vi "Z6_Beamline.Calc BL State.vi"(0 "i ref in":refnum<vi>, 5 "error in (nop error)":errorcluster) -> (14 "i ref out":refnum<vi>, 19 "error out":errorcluster)   [LabVIEW 2014, in "Z6_Beamline.lvlib"]
doc: "this VI calculates the global state of the beamline, writes the result to own attributes, and publishes it as service."
uses:
  Z6_Beamline.lvlib
  PH_BL-Master/PH_BL-Master.lvlib
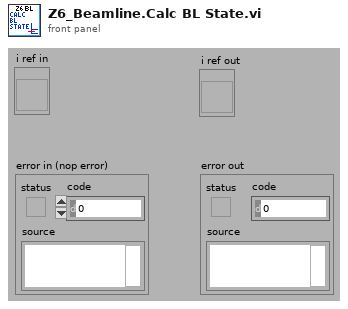
[diagram p1: front panel]
types:
  T1 = typedef "Z6_Beamline.lvlib/Z6_Beamline.i attribute.ctl" = cluster{"Subs ok GUI Refs":T2, "Refs BL Northtower":refnum<vi>[], "Refs BL Southtower":refnum<vi>[], "Refs BL 100TW COS":refnum<vi>[], "State Subsystems":cluster{"Northtower":bool, "Southtower":bool, "Frontends":bool, "100TW COS":bool}, "Z6 Beamline Status Subscriber Information":T3, "Color State PHELIX":i16}
  T2 = typedef "Z6_Beamline.lvlib/Z6_Beamline.Subsystem ok GUI Refs.ctl" = cluster{"Northtower ok":refnum<vi>, "Southtower ok":refnum<vi>, "Frontends ok":refnum<vi>, "100TW COS ok":refnum<vi>}
  T3 = typedef "Z6_Beamline.lvlib/Z6_Beamline.Status Subscriber Information.ctl" = cluster{"BL Z6 Shutter":T4, "CH 10":T4, "CH 11":T4, "ST Flip Cam":T4, "ST Flip DB":T4, "BL Z6 Dump":T4}
  T4 = typedef "PH_BL-Master.lvlib/PH_BL-Master.Status Subscriber Information.ctl" = cluster{"Index of element":i32, "Attributeset":T5}
  T5 = typedef "PH_BL-Master.lvlib/PH_BL-Master.Attribute Set.ctl" = enum16{"Boolean Status Service Subscriber", "Picture Status Service Subscriber"}
  T6 = cluster{"Northtower":bool, "Southtower":bool, "Frontends":bool, "100TW COS":bool}
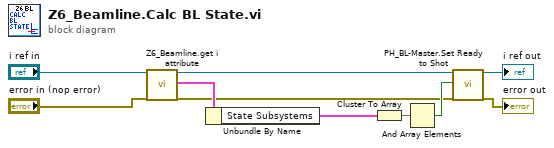
[diagram p0: block diagram]
diagram:
  n1 = call "Z6_Beamline.get i attribute.vi"("i ref in"="i ref in", "error in (no error)"="error in (nop error)") -> ("i ref out"=w4:refnum<vi>, "i attribute"=w10:T1, "error out"=w1:errorcluster)  [unwired: 15 in]
  n2 = Unbundle By Name(w10) -> ("State Subsystems"=w8:T6)
  n3 = Cluster To Array(cluster=w8) -> (array=w9:bool[])
  n4 = And Array Elements(Boolean array=w9) -> (logical AND=w5:bool)
  n5 = call "PH_BL-Master.Set Ready to Shot.vi"("i ref in"=w4, "R2S?"=w5, "error in (no error)"=w1) -> ("i ref out"=→"i ref out":refnum<vi>, "error out"=→"error out":errorcluster)  [unwired: 15 in]
